vi "sv_Align Waveforms by Leading Sync Pulse_Copy.vi"(6 "maximum delay":i32=51200, 7 "reset":bool, 8 "error in (no error)":errorcluster, 10 "response signals":waveform(dbl)[](array[waveform]), 11 "alignment reference signal":waveform(dbl)={"t0"=timestamp(0 s since 1904-01-01), "dt"=0.0, "Y"=[]}) -> (0 "error out":errorcluster, 1 "residual delays [s]":dbl[](array[numeric]) format="%.2p", 2 "aligned signals":waveform(dbl)[](array[waveform]), 4 "aligned signals length":i32, 5 "alignment reference detected":bool)   [LabVIEW 2021, in "Audio ADC Shared.lvlib"]
doc: "Use this VI to measure the delay from reference to each response and effectively remove the integer sample delay on each channel in order to align the responses according to expected reference signal."
uses:
  Audio ADC Shared.lvlib
  <vilib>/addons/Sound and Vibration/svt_Calibration/SV Measure Delay and Polarity and Coherence (Nx1).vi
  Program Files/National Instruments/LabVIEW 2021/examples/Sound and Vibration/Audio Measurements/subVIs/sv_Assign Delay to Idle Channels.vi
  <vilib>/addons/_NISVFA/_Shared subVIs/Common/svc_Check for Waveform Parameter Continuity (N Ch).vi
  <vilib>/addons/Sound and Vibration/svt_Calibration/SV Measure Delay and Polarity and Coherence.vi
  <vilib>/addons/_NISVFA/_Shared subVIs/Common/sv_Get NI Property Name String.vi
  <vilib>/addons/_NISVFA/_Shared subVIs/Common/svc_Check for Waveform Parameter Continuity (no state).vi
  <vilib>/Analysis/_algsub.llb/Vector Norm.vi
  <vilib>/Analysis/_algsub.llb/Real Vector Norm.vi
  <vilib>/addons/_NISVFA/_Shared subVIs/Common/SV Get Data Subset.vi
  <vilib>/addons/_NISVFA/_Shared subVIs/Common/svc_Get Array Subset (Index).vi
  <vilib>/addons/_NISVFA/_Shared subVIs/Common/svc_Get SV Channel Info.vi
  <vilib>/addons/_NISVFA/_Shared subVIs/Common/svc_Coerce Index and Length.vi
  <vilib>/addons/_NISVFA/_Shared subVIs/Common/svc_Unit Label to Engineering Units.vi
  <vilib>/addons/_NISVFA/_Shared subVIs/Common/svc_Engineering Units to Unit Label.vi
  <vilib>/addons/_NISVFA/_Shared subVIs/Common/svc_Conditional Merge Error.vi
  <vilib>/addons/_NISVFA/_Shared subVIs/Data Objects/Waveforms (DBL)/SV Read Newest Data.vi
  <vilib>/measure/maresamp.llb/Resample Waveforms (single shot).vi
  <vilib>/measure/maresamp.llb/Resample Waveform (single shot).vi
  <vilib>/addons/_NISVFA/_Shared subVIs/Common/svc_Check dt for Equal Sample Rates.vi
  <vilib>/Waveform/TSOps.llb/Timestamp Subtract.vi
  <vilib>/Analysis/2dsp.llb/CrossCorrelation.vi
  <vilib>/Analysis/2dsp.llb/1D Cross Correlation (DBL).vi
  <vilib>/addons/_NISVFA/_Shared subVIs/Common/svc_Fit Quadratic to Max Three Points in Array.vi
  <vilib>/Utility/error.llb/Error Cluster From Error Code.vi
  <vilib>/addons/_NISVFA/_Shared subVIs/Common/svc_Caller VI Returned in Error Source.vi
  <vilib>/addons/_NISVFA/_Shared subVIs/Data Objects/Waveforms (DBL)/Waveforms (N Ch).lvclass
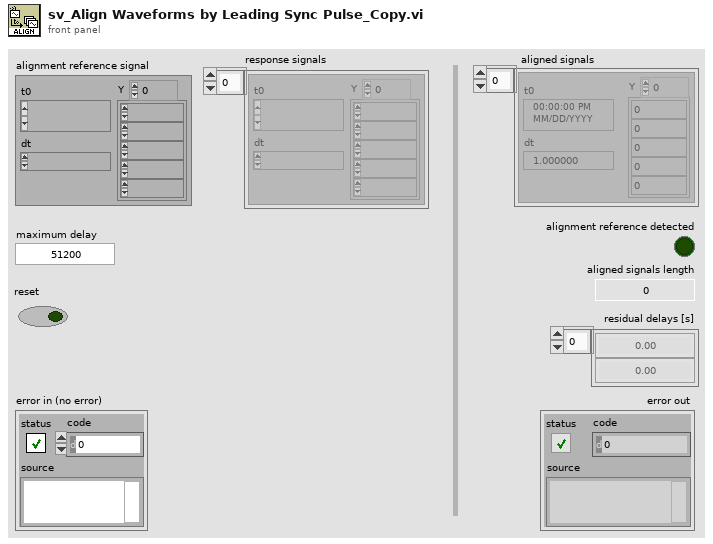
[diagram p1: front panel]
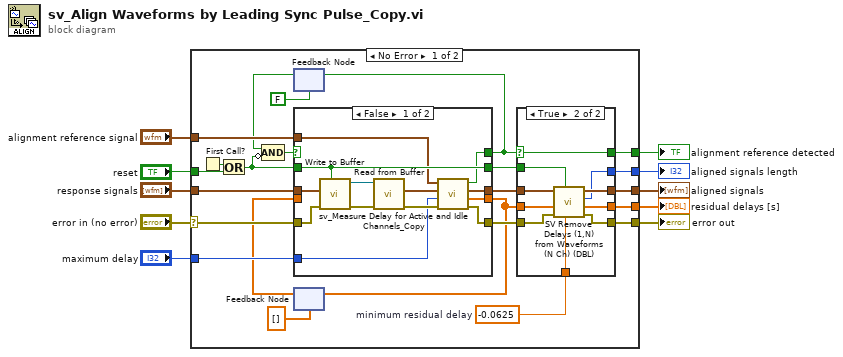
[diagram p0: block diagram]
diagram:
  n1 = case shown="No Error" "error in (no error)" {
    selector: "error in (no error)" -> [w30 w65]
    tunnel: "response signals" -> [w33 _]
    tunnel: "alignment reference signal" -> [w32 _]
    tunnel: "maximum delay" -> [w31 _]
    tunnel: [w12 _] -> w6
    tunnel: [w25 _] -> w5
    tunnel: [w24 _] -> w4
    tunnel: [w23 _] -> w3
    tunnel: "reset" -> [w17 _]
    tunnel: [w13 w65] -> w1
    frame No Error {
      w11 = -0.0625  # minimum residual delay
      n2 = First Call?() -> (First Call?: T/F=w18:bool)
      n3 = Or(x=w18, y=w17) -> (x .or. y?=w16:bool)
      n4 = feedback #1(FALSE) -> (w15:bool)
      n5 = Compound Arithmetic op=AND(w15, invert w16) -> (w14:bool)
      n6 = feedback #2(dbl[] [] ("Array")) -> (w20:dbl[])
      n7 = case shown="False" w14 {
        selector: w14 -> [_ w50]
        tunnel: w33 -> [w43 w51]
        tunnel: w32 -> [w37 _]
        tunnel: w31 -> [w36 _]
        tunnel: w30 -> [w46 w49]
        tunnel: [w44 w49] -> w29
        tunnel: [w34 w51] -> w28
        tunnel: [w35 w50] -> w27
        tunnel: [w39 w48] -> w21
        tunnel: w20 -> [_ w48]
        tunnel: w16 -> [w45 w47]
        tunnel: [w45 w47] -> w19
        frame False {
          n8 = call <vilib>:"Write to Buffer.vi"("clear buffer (False)"=w45, "error in (no error)"=w46, "waveforms"=w43) -> ("error out"=w41:errorcluster, "buffer out"=w42:refnum<data-value>)  [unwired: 6 in, 1 out]
          n9 = call-poly <vilib>:"Read from Buffer.vi"("error in (no error)"=w41, "buffer"=w42) -> ("error out"=w40:errorcluster, "waveforms subset"=w38:waveform(dbl)[])  [unwired: 6 in, 2 out]
          n10 = call "sv_Measure Delay for Active and Idle Channels_Copy.vi"("error in (no error)"=w40, "maximum delay"=w36, "waveforms subset"=w38, "alignment reference signal"=w37) -> ("error out"=w44:errorcluster, "delays [s]"=w39:dbl[], "waveforms subset dup"=w34:waveform(dbl)[], "reference detected"=w35:bool)  [unwired: 4 in]
        }
        frame True {
        }
      }
      n11 = feedback-in #1(w27) -> ()
      n12 = feedback-in #2(w21) -> ()
      n13 = case shown="True" w27 {
        selector: w27 -> [w53 w56]
        tunnel: w29 -> [w54 w64]
        tunnel: w28 -> [w52 w63]
        tunnel: w19 -> [_ w62]
        tunnel: w21 -> [_ w60]
        tunnel: [w52 w61] -> w25
        tunnel: [_ w59] -> w24
        tunnel: [_ w58] -> w23
        tunnel: [w54 w57] -> w13
        tunnel: [w53 w56] -> w12
        tunnel: w11 -> [_ w55]
        frame False {
        }
        frame True {
          n14 = call <vilib>:"SV Remove Delays (1,N) from Waveforms (N Ch) (DBL).vi"("minimum residual delay"=w55, "reset"=w62, "error in (no error)"=w64, "path-dependent analog delays [s]"=w60, "scaled signals"=w63) -> ("error out"=w57:errorcluster, "residual delays [s]"=w58:dbl[], "aligned signals length"=w59:i32, "aligned signals"=w61:waveform(dbl)[])  [unwired: 3 in]
        }
      }
    }
    frame Error {
    }
  }
  "aligned signals" <- w5
  "alignment reference detected" <- w6
  "aligned signals length" <- w4
  "residual delays [s]" <- w3
  "error out" <- w1
